vi "phase_correct_coupling.vi"(4 "Really correct?":bool=TRUE, 6 "Is low?":bool, 10 "Complex coupling":cdb[][](array[numeric]) format="%#.3f", 11 "Ref carrier ampl":cdb[][][](array[numeric]) format="%#.3f") -> (2 "Phase corrected coupling":cdb[][](array[numeric]) format="%#.3f", 3 "Phase mismatch":dbl[][](array[numeric]) format="%#.3f")   [LabVIEW 2014]
panel:
  out "Ref magnitude":dbl[][](array[numeric]) format="%#.3f"
  out "Ref phase":dbl[][](array[numeric]) format="%#.3f"
  # "Amplitudes for the selected card"
  # "Is this a low rate coupling?"
  # "If false, don't actually do anything, just pass coupling through."
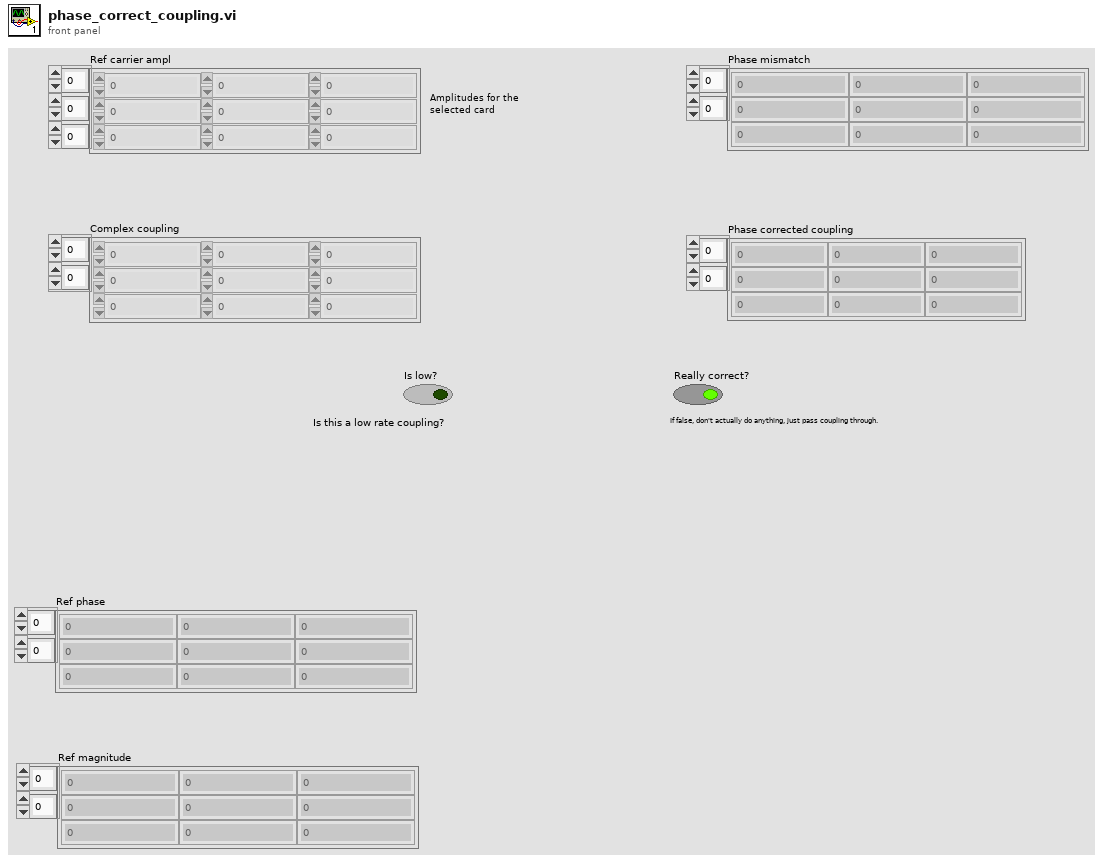
[diagram p1: front panel]
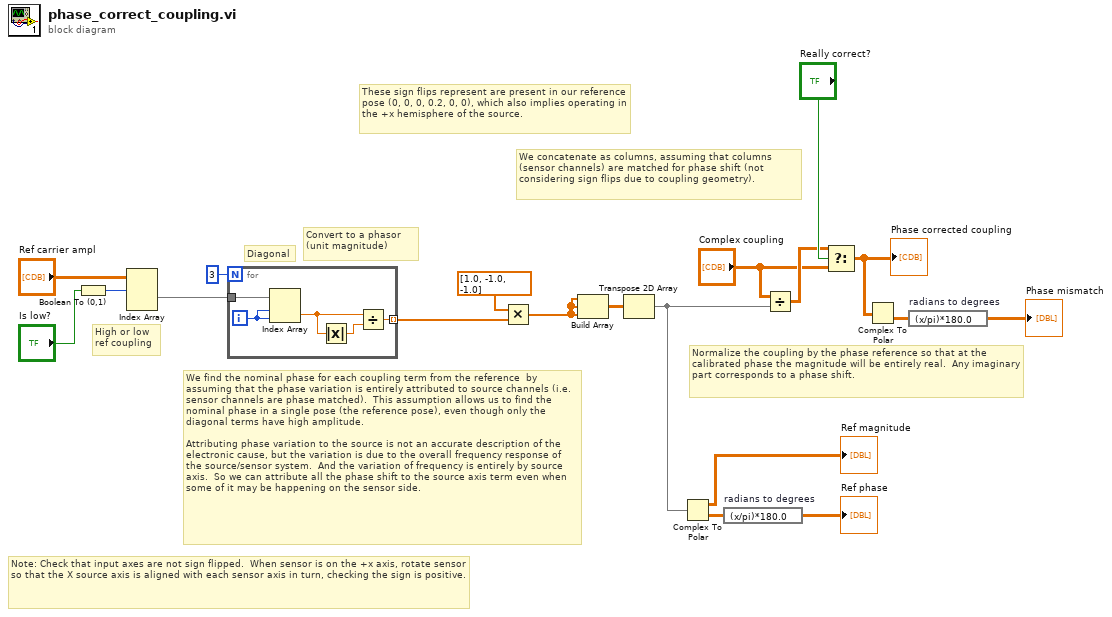
[diagram p0: block diagram]
diagram:
  # "High or low\nref coupling"
  # "Note: Check that input axes are not sign flipped.  When sensor is on the +x axis, rotate sensor so that the X source axis is aligned with each sensor axis in turn, checking the sign is positive."
  # "These sign flips represent are present in our reference pose (0, 0, 0, 0.2, 0, 0), which also implies operating in the +x hemisphere of the source."
  # "Normalize the coupling by the phase reference so that at the calibrated phase the magnitude will be entirely real.  Any imaginary part corresponds to a phase shift."
  # "We concatenate as columns, assuming that columns (sensor channels) are matched for phase shift (not considering sign flips due to coupling geometry)."
  # "Convert to a phasor (unit magnitude)"
  # "Diagonal"
  # "We find the nominal phase for each coupling term from the reference  by assuming that the phase variation is entirely attributed to source channels (i.e. sensor channels are phase matched).  This assumption allows us to find the nominal phase in a single pose (the reference pose), even though only the diagonal terms have high amplitude. \n\nAttributing phase variation to the source is not an accurate description of the electronic cause, but the variation is due to the overall frequency response of the source/sensor system.  And the variation of frequency is entirely by source axis.  So we can attribute all the phase shift to the source axis term even when some of it may be happening on the sensor side."
  n1 = Boolean To (0,1)(Boolean="Is low?") -> (0, 1=w2:i16)
  n2 = Index Array(array="Ref carrier ampl", index (dim 0)=w2) -> (element=w1:cdb[][])  [unwired: 2 in]
  n3 = for {
    N: 3 -> [_]
    tunnel: w1 -> [w24]
    tunnel: [w20] -> w13 mode=indexing
    i -> [w23]
    n4 = Index Array(array=w24, index (row)=w23, index (col)=w23) -> (element=w21:cdb)
    n5 = Absolute Value(x=w21) -> (abs(x)=w22:dbl)
    n6 = Divide(x=w21, y=w22) -> (x/y=w20:cdb)
  }
  n7 = Multiply(x=dbl[] [1.0, -1.0, -1.0] ("Sign flips"), y=w13) -> (x*y=w10:cdb[])
  n8 = Build Array(w10, w10, w10) -> (w8:cdb[][])
  n9 = Transpose 2D Array(2D array=w8) -> (transposed array=w7:cdb[][])
  n10 = Complex To Polar(r * e^(i*theta)=w7) -> (r=→"Ref magnitude":dbl[][], theta=w11:dbl[][])
  n11 = expression code="(x/pi)*180.0" "radians to degrees"(w11) -> (→"Ref phase":dbl[][])
  n12 = Divide(x="Complex coupling", y=w7) -> (x/y=w5:cdb[][])
  n13 = Select(t=w5, s="Really correct?", f="Complex coupling") -> (s? t:f=w3:cdb[][])
  "Phase corrected coupling" <- w3
  n14 = Complex To Polar(r * e^(i*theta)=w3) -> (theta=w16:dbl[][])  [unwired: 1 out]
  n15 = expression code="(x/pi)*180.0" "radians to degrees"(w16) -> (→"Phase mismatch":dbl[][])
